vi "Write Multi U64.vi"(8 "error in (no error)":errorcluster, 9 "U64's":u64[](array[numeric]), 10 "Tag":string[](array[string]), 11 "Omni_Bus in":refnum<class "Omni_Bus.lvclass">) -> (0 "error out":errorcluster, 3 "Omni_Bus out":refnum<class "Omni_Bus.lvclass">)   [LabVIEW 2021, in "Omni_Bus.lvclass"]
uses:
  Omni_Bus.lvclass
  <vilib>/TSA/Abstract Data Classes/Abs_Types/U64 Integer/Abs_U64 Integer.lvclass
  C:/Program Files (x86)/National Instruments/LabVIEW 2021/vi.lib/TSA/Abstract Data Classes/Abs_Types/Type/Abs_Type.lvclass
  <vilib>/TSA/Abstract Data Classes/Abs_Types/Type/Abs_Type.lvclass/Abs_Type.ctl
  Omni_Bus.lvclass/Omni_Bus.ctl
  FindMultiVar.vi
  FindVar.vi
  <vilib>/Utility/error.llb/Clear Errors.vi
  Properties/Read Var Map.vi
  <vilib>/TSA/Abstract Data Classes/Abs_Types/Type/Properties/Read Tag.vi
  <vilib>/TSA/Abstract Data Classes/Abs_Types/Value/Abs_Value.lvclass
  Check For Read Only Error.vi
  Incorrect Tag String Error.vi
  <vilib>/TSA/Abstract Data Classes/Abs_Types/Type/Abs_Type.lvclass
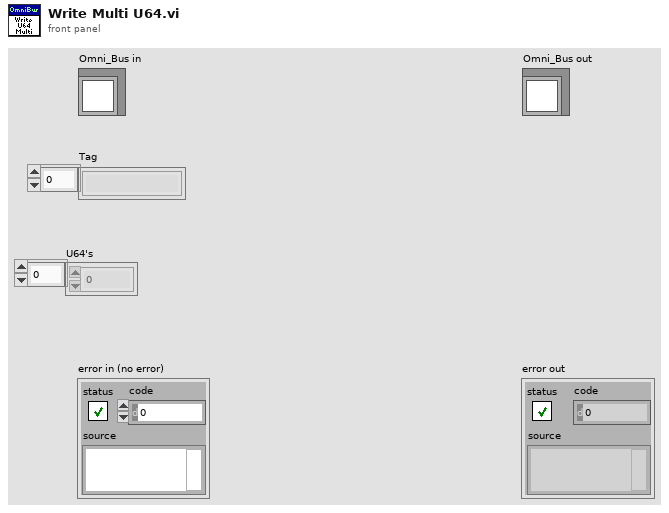
[diagram p1: front panel]
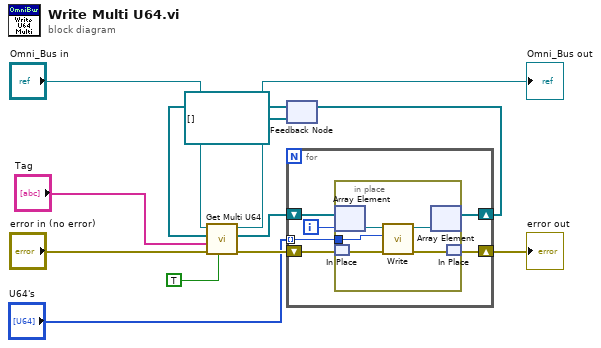
[diagram p0: block diagram]
diagram:
  n1 = feedback #1(refnum<class "Abs_U64 Integer.lvclass">[] [] ("Value Out")) -> (w8:refnum<class "Abs_U64 Integer.lvclass">[])
  n2 = call "Get Multi U64.vi"("Write?"=TRUE, "error in (no error)"="error in (no error)", "Tag"="Tag", "Value Type"=w8, "Var Bus in"="Omni_Bus in") -> ("error out"=w6:errorcluster, "Value Out"=w5:refnum<class "Abs_U64 Integer.lvclass">[], "Var Bus out"=→"Omni_Bus out":refnum<class "Omni_Bus.lvclass">)  [unwired: 3 in, 1 out]
  n3 = for {
    tunnel: "U64's" -> [w18] mode=indexing
    shift-right: [w13] -> w2
    shift-left: w6 -> [w14]
    shift-right: [w16] -> w3
    shift-left: w5 -> [w17]
    i -> [w15]
    n4 = in-place {
      in-place-border: w18 -> [w23]
      n5 = in-place-array #2(w17, w15) -> (w22:refnum<class "Abs_U64 Integer.lvclass">)
      n6 = in-place-match #3(w14) -> (w20:errorcluster)
      n7 = call-dynamic "Write.vi"("error in (no error)"=w20, "Value"=w23, "Double Float.lvclass_340760 in"=w22) -> ("error out"=w19:errorcluster, "Double Float.lvclass_340760 out"=w21:refnum<class "Abs_U64 Integer.lvclass">)  [unwired: 7 in]
      n8 = in-place-array #2(w21) -> (w16:refnum<class "Abs_U64 Integer.lvclass">[])  [unwired: 1 out]
      n9 = in-place-match #3(w19) -> (w13:errorcluster)
    }
  }
  "error out" <- w2
  n10 = feedback-in #1(w3) -> ()
